vi "CompareArrays.vi"(4 "indexed loaded Array":dbl[][](array[numeric]), 5 "Name Array":string[](array[string]), 7 "DIMControSet":refnum<vi>[](array[refnum])) -> (2 "Table for loading values":string[][](array[string]) caption="Test.set")   [LabVIEW 2014, in "Panels.lvlib"]
uses:
  Panels.lvlib
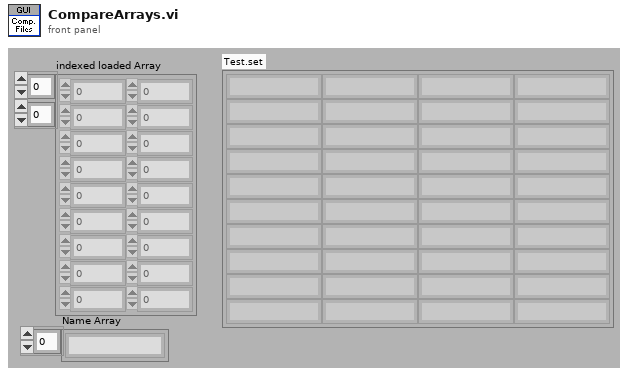
[diagram p1: front panel]
types:
  T1 = cluster{"data":dbl[], "no link":bool, "quality":i32, "timeStamp":dbl}
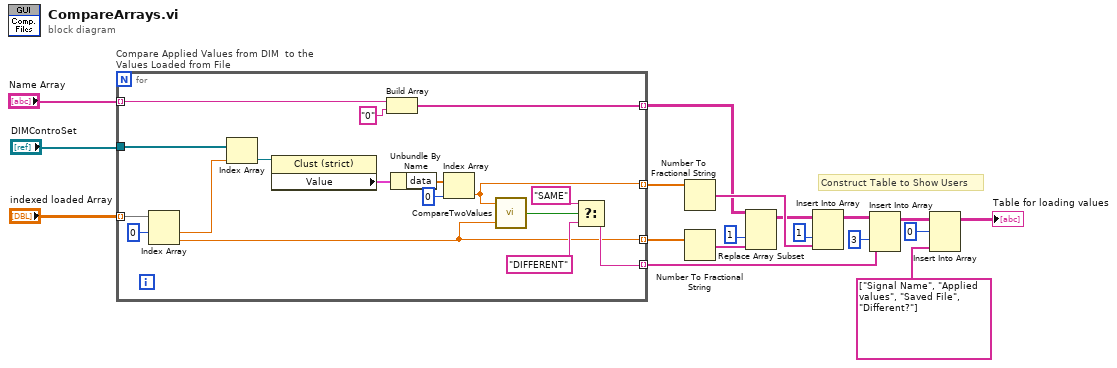
[diagram p0: block diagram]
diagram:
  # "Construct Table to Show Users"
  n1 = for "Compare Applied Values from DIM  to the Values Loaded from File" {
    tunnel: "indexed loaded Array" -> [w32] mode=indexing
    tunnel: [w27] -> w8 mode=indexing
    tunnel: [w24] -> w14 mode=indexing
    tunnel: [w33] -> w18 mode=indexing
    tunnel: "DIMControSet" -> [w23]
    tunnel: [w30] -> w5 mode=indexing
    tunnel: "Name Array" -> [w20] mode=indexing
    n2 = Index Array(array=w32, index #1=0 ("index")) -> (element #1=w19:dbl, element #2=w24:dbl)  [unwired: 1 in]
    n3 = Index Array(array=w23, index=w19) -> (element=w21:refnum<vi>)
    n4 = property class="Clust (strict)"(reference=w21) -> ("Value"=w22:T1)  [unwired: 1 in, 2 out]
    n5 = Build Array(w20, "0" ("element")) -> (w30:string[])
    n6 = Unbundle By Name(w22) -> ("data"=w28:dbl[])
    n7 = Index Array(array=w28, index=0) -> (element=w27:dbl)
    n8 = call "CompareTwoValues.vi"("number2"=w24, "number1"=w27) -> ("x < y?"=w26:bool)
    n9 = Select(t="SAME", s=w26, f="DIFFERENT") -> (s? t:f=w33:string)
  }
  n10 = Number To Fractional String(number=w8) -> (F-format string=w10:string[])  [unwired: 3 in]
  n11 = Number To Fractional String(number=w14) -> (F-format string=w4:string[])  [unwired: 3 in]
  n12 = Replace Array Subset(array=w5, new element=w4, index (col)=1 ("disabled index (col)")) -> (w3:string[][])  [unwired: 1 in]
  n13 = Insert Into Array(array=w3, index (col)=1 ("disabled index (col)"), new element=w10) -> (w15:string[][])  [unwired: 1 in]
  n14 = Insert Into Array(array=w15, index (col)=3 ("disabled index (col)"), new element=w18) -> (w16:string[][])  [unwired: 1 in]
  n15 = Insert Into Array(array=w16, index (row)=0, new element=string[] ["Signal Name", "Applied values", "Saved File", "Different?"]) -> (→"Table for loading values":string[][])  [unwired: 1 in]
